vi "Initialize Steering Frame.vi"(6 "wheel frame angles (rad)":dbl[](array[numeric]), 7 "wheels":refnum<class "NI_Robotics_Wheel.lvclass">[](array[class]), 8 "error in (no error)":errorcluster, 9 "wheel y positions":dbl[](array[numeric]), 10 "wheel x positions":dbl[](array[numeric]), 11 "steering frame in":refnum<class "NI_Robotics_Steering Frame.lvclass">) -> (0 "error out":errorcluster, 3 "steering frame out":refnum<class "NI_Robotics_Steering Frame.lvclass">)   [LabVIEW 2017, in "NI_Robotics_Steering Frame.lvclass"]
uses:
  <vilib>/robotics/Steering/Steering Frame/NI_Robotics_Steering Frame.lvclass
  <vilib>/robotics/Steering/Wheel/NI_Robotics_Wheel.lvclass
  <vilib>/robotics/Steering/Wheel/Wheel State.ctl
  <vilib>/robotics/Steering/Steering Frame/Wheel Orientation.ctl
  <vilib>/robotics/Steering/Wheel/NI_Robotics_Wheel.lvclass/NI_Robotics_Wheel.ctl
  <vilib>/robotics/Steering/Steering Frame/NI_Robotics_Steering Frame.lvclass/NI_Robotics_Steering Frame.ctl
  <vilib>/Analysis/coordinate.llb/Wrap Angle (array).vi
  <vilib>/Analysis/NI_AAL_Angle.lvlib
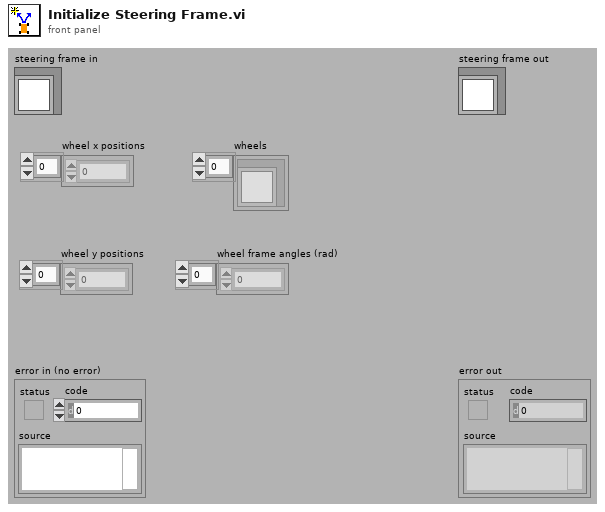
[diagram p1: front panel]
types:
  T1 = typedef "NI_Robotics_Steering Frame.lvclass/Wheel Orientation.ctl" = cluster{"wheel":refnum<class "NI_Robotics_Wheel.lvclass">, "x position":dbl, "y position":dbl, "frame angle (rad)":dbl}
  T2 = typedef "NI_Robotics_Wheel.lvclass/Wheel State.ctl" = cluster{"wheel name":string, "forward angular velocity":dbl, "caster angular velocity":dbl, "caster wheel angle (rad)":dbl, "steering angle (rad)":dbl}
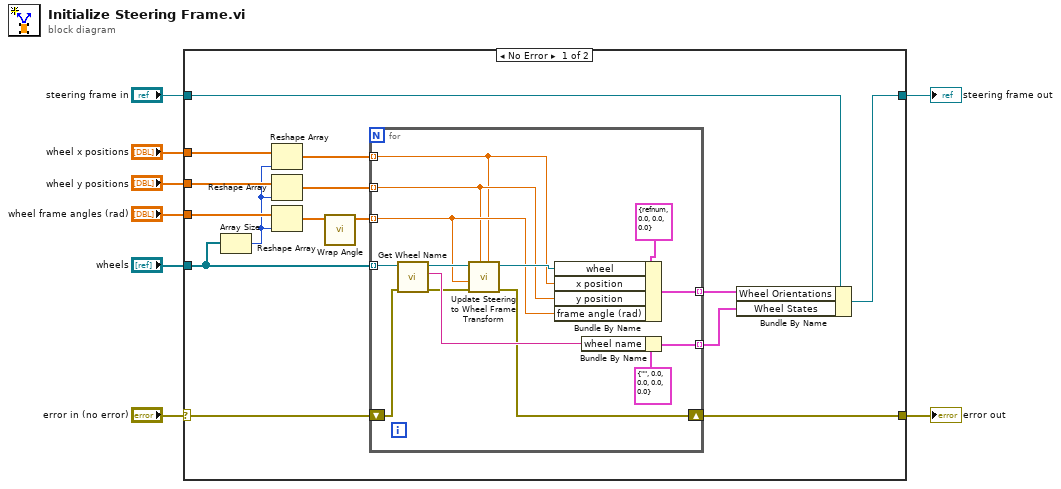
[diagram p0: block diagram]
diagram:
  n1 = case shown="No Error" "error in (no error)" {
    selector: "error in (no error)" -> [w12 w39]
    tunnel: [w11 w39] -> w7
    tunnel: [w15 w38] -> w5
    tunnel: "steering frame in" -> [w17 w38]
    tunnel: "wheels" -> [w20 _]
    tunnel: "wheel x positions" -> [w23 _]
    tunnel: "wheel y positions" -> [w22 _]
    tunnel: "wheel frame angles (rad)" -> [w21 _]
    frame No Error {
      n2 = Array Size(array=w20) -> (size(s)=w14:i32)
      n3 = Reshape Array(w23, w14) -> (w19:dbl[])
      n4 = Reshape Array(w22, w14) -> (w18:dbl[])
      n5 = Reshape Array(w21, w14) -> (w10:dbl[])
      n6 = call-poly <vilib>:"Wrap Angle.vi"("Angle In"=w10) -> ("Angle Out"=w9:dbl[])  [unwired: 9 in, 1 out]
      n7 = for {
        tunnel: w20 -> [w37] mode=indexing
        tunnel: w19 -> [w24] mode=indexing
        tunnel: w18 -> [w25] mode=indexing
        tunnel: w9 -> [w26] mode=indexing
        shift-right: [w27] -> w11
        shift-left: w12 -> [w35]
        tunnel: [w33] -> w13 mode=indexing
        tunnel: [w31] -> w16 mode=indexing
        n8 = call <vilib>:"Get Wheel Name.vi"("error in (no error)"=w35, "wheel in"=w37) -> ("error out"=w28:errorcluster, "wheel name"=w36:string, "wheel out"=w30:refnum<class "NI_Robotics_Wheel.lvclass">)  [unwired: 7 in]
        n9 = call <vilib>:"Update Steering to Wheel Frame Transform.vi"("x wheel position"=w24, "y wheel position"=w25, "error in (no error)"=w28, "wheel frame angle (rad)"=w26, "wheel in"=w30) -> ("error out"=w27:errorcluster, "wheel out"=w29:refnum<class "NI_Robotics_Wheel.lvclass">)  [unwired: 5 in]
        n10 = Bundle By Name(cluster=T1 {"wheel"=refnum, "x position"=0.0, "y position"=0.0, "frame angle (rad)"=0.0} ("Wheel Orientation"), "wheel"=w29, "x position"=w24, "y position"=w25, "frame angle (rad)"=w26) -> (w31:T1)
        n11 = Bundle By Name(cluster=T2 {"wheel name"="", "forward angular velocity"=0.0, "caster angular velocity"=0.0, "caster wheel angle (rad)"=0.0, "steering angle (rad)"=0.0} ("wheel state"), "wheel name"=w36) -> (w33:T2)
      }
      n12 = Bundle By Name(cluster=w17, "Wheel Orientations"=w16, "Wheel States"=w13) -> (w15:refnum<class "NI_Robotics_Steering Frame.lvclass">)
    }
    frame Error {
    }
  }
  "error out" <- w7
  "steering frame out" <- w5
